vi "Read Fault List.vi"(8 "error in":errorcluster, 9 "timeout (-1)":i32=-1, 11 "Engine Runtime Interface in":refnum<class "Engine Runtime Interface.lvclass">) -> (0 "error out":errorcluster, 2 "faults":T1[](array[typedef]), 3 "Engine Runtime Interface out":refnum<class "Engine Runtime Interface.lvclass">)   [LabVIEW 2013, in "Engine Runtime Interface.lvclass"]
doc: "Retrieves all uncleared faults from the engine. Faults are any recoverable errors which did not result in engine shutdown."
uses:
  Engine Runtime Interface.lvclass
  Fault.ctl
  <vilib>/NI/Tag Bus Module Framework/runtime/error classification.ctl
  <vilib>/NI/Configuration Framework/NISE_CEF_TreeControl.lvlib
  <vilib>/NI/Tag Bus Module Framework/runtime/TBM module execution interface.lvclass
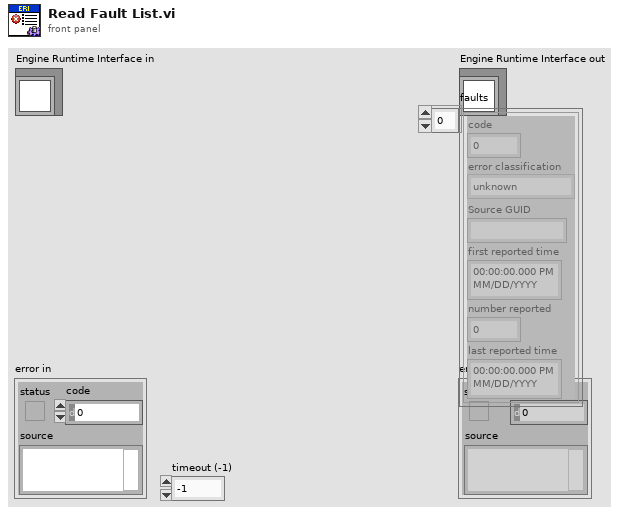
[diagram p1: front panel]
types:
  T1 = typedef "Engine Runtime Interface.lvclass/Fault.ctl" = cluster{"code":i32, "error classification":T2, "Source GUID":string, "first reported time":timestamp, "number reported":u32, "last reported time":timestamp}
  T2 = typedef "TBM module execution interface.lvclass/error classification.ctl" = enum16{"unknown", "none", "trivial", "recoverable", "critical"}
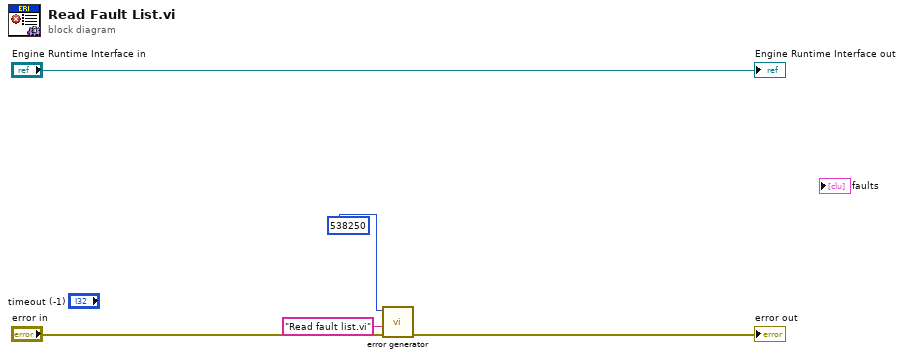
[diagram p0: block diagram]
diagram:
  n1 = call <vilib>:"error generator.vi"("error in"="error in", "source"="Read fault list.vi", "error code (0)"=538250) -> ("error out"=→"error out":errorcluster)  [unwired: 6 in]
  "Engine Runtime Interface out" <- "Engine Runtime Interface in"
